vi "Shift_Block.vi"(8 "y":dbl, 9 "x":dbl, 11 "old":T1 {"orientaion" items=["up", "down", "left", "right"]; "type" items=["t", "rl", "ll", "rz", "lz", "square", "line"]}) -> (3 "new":T1 {"orientaion" items=["up", "down", "left", "right"]; "type" items=["t", "rl", "ll", "rz", "lz", "square", "line"]})   [LabVIEW 2015]
uses:
  block.ctl
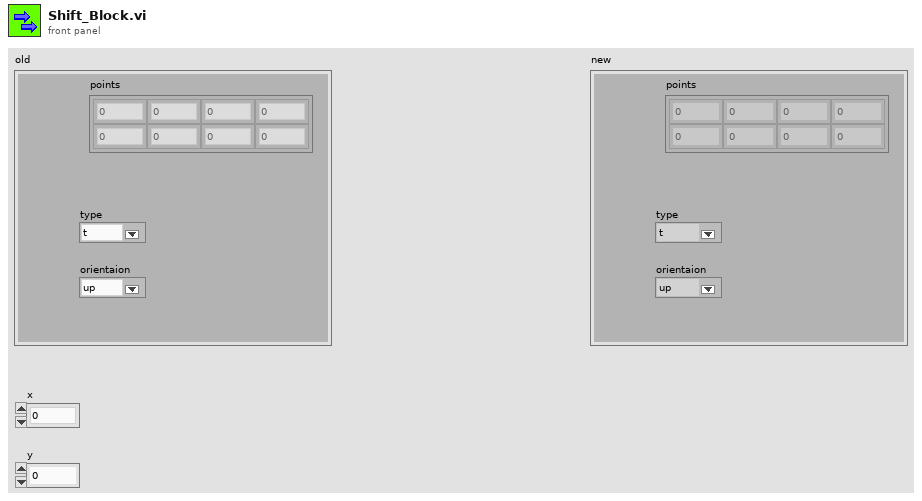
[diagram p1: front panel]
types:
  T1 = typedef "block.ctl" = cluster{"points":dbl[][], "type":u16, "orientaion":u16}
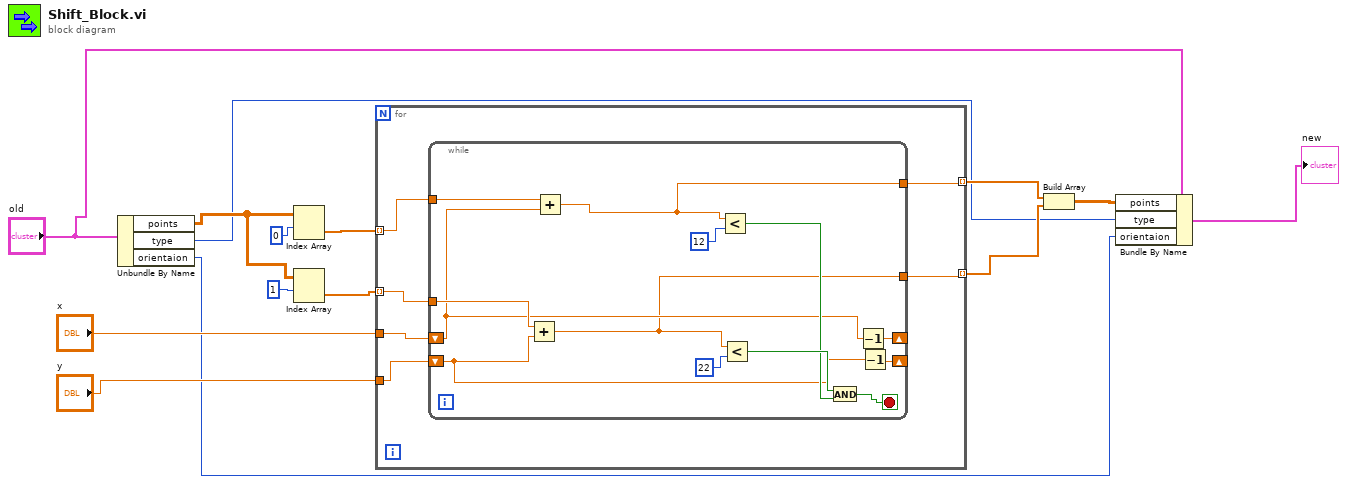
[diagram p0: block diagram]
diagram:
  n1 = Unbundle By Name("old") -> ("points"=w12:dbl[][], "type"=w3:u16, "orientaion"=w2:u16)
  n2 = Index Array(array=w12, index (row)=0) -> (element=w11:dbl[])  [unwired: 1 in]
  n3 = Index Array(array=w12, index (row)=1) -> (element=w10:dbl[])  [unwired: 1 in]
  n4 = for {
    tunnel: w11 -> [w20] mode=indexing
    tunnel: w10 -> [w19] mode=indexing
    tunnel: "x" -> [w18]
    tunnel: "y" -> [w17]
    tunnel: [w16] -> w6 mode=indexing
    tunnel: [w15] -> w7 mode=indexing
    n5 = while {
      tunnel: w20 -> [w33]
      tunnel: w19 -> [w32]
      shift-right: [w25] -> _
      shift-left: w17 -> [w23]
      shift-right: [w26] -> _
      shift-left: w18 -> [w24]
      tunnel: [w22] -> w16
      tunnel: [w21] -> w15
      stop <- w31 stop-if-true
      n6 = Add(x=w32, y=w23) -> (x+y=w21:dbl)
      n7 = Add(x=w33, y=w24) -> (x+y=w22:dbl)
      n8 = Less?(x=w22, y=12) -> (x < y?=w27:bool)
      n9 = Less?(x=w21, y=22) -> (x < y?=w28:bool)
      n10 = And(x=w28, y=w27) -> (x .and. y?=w31:bool)
      n11 = Decrement(x=w24) -> (x-1=w26:dbl)
      n12 = Decrement(x=w23) -> (x-1=w25:dbl)
    }
  }
  n13 = Build Array(w6, w7) -> (w4:dbl[][])
  n14 = Bundle By Name(cluster="old", "points"=w4, "type"=w3, "orientaion"=w2) -> (→"new":T1)
